vi "Set ATP ComboBox - Single Project Open.vi"(8 "Error In":errorcluster, 10 "Project Name":string, 11 "Project Name ComboBox Ref":refnum<vi>) -> (0 "Error Out":errorcluster)   [LabVIEW 2022 SP3]
doc: "ATP = \"Add to Project?\" drop-down menu"
uses:
  <vilib>/Utility/miscctls.llb/LVFontTypeDef.ctl
panel:
  # "Development\nControls or indicators that are useful for development or testing, but which are not outputs of the VI."
  # "Input\nInputs to the VI"
  # "Output\nOutputs of the VI"
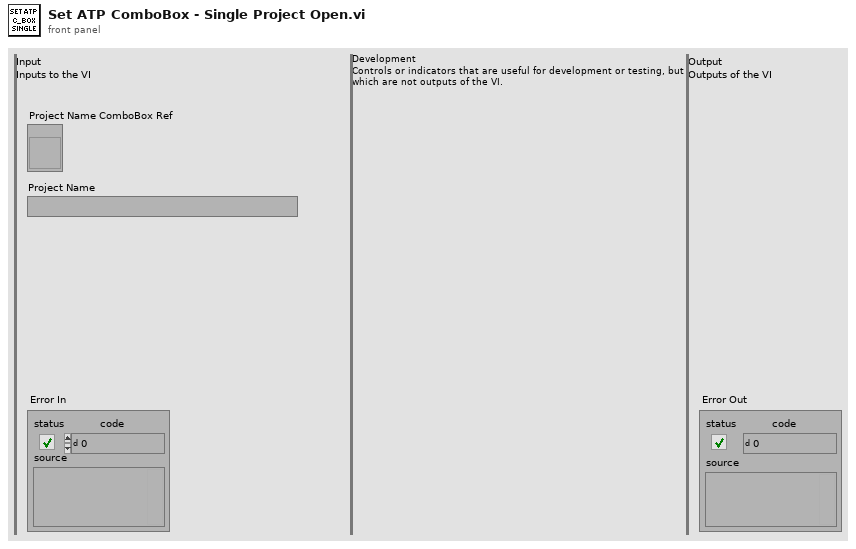
[diagram p1: front panel]
types:
  T1 = typedef "LVFontTypeDef.ctl" = cluster{"Font Name":string, "Size":u16, "Bold":bool, "Italic":bool, "Underline":bool, "Strikeout":bool, "Color":u32}
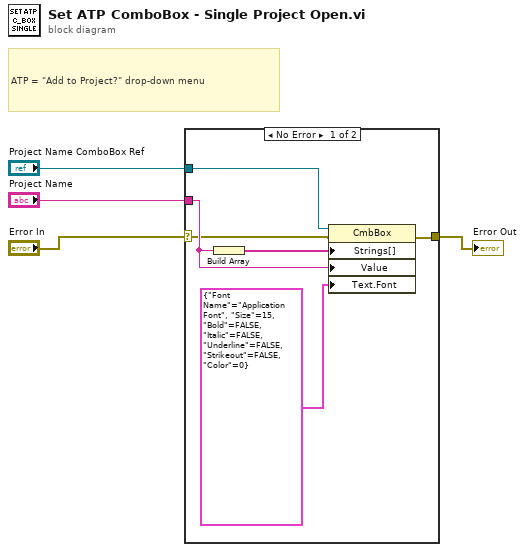
[diagram p0: block diagram]
diagram:
  # "ATP = \"Add to Project?\" drop-down menu"
  n1 = case shown="No Error" "Error In" {
    selector: "Error In" -> [w7 w11]
    tunnel: [w6 w11] -> w3
    tunnel: "Project Name ComboBox Ref" -> [w9 _]
    tunnel: "Project Name" -> [w8 _]
    frame No Error {
      n2 = Build Array(w8) -> (w5:string[])
      n3 = property class="CmbBox"(reference=w9, error in=w7, "Strings[]"=w5, "Value"=w8, "Text.Font"=T1 {"Font Name"="Application Font", "Size"=15, "Bold"=FALSE, "Italic"=FALSE, "Underline"=FALSE, "Strikeout"=FALSE, "Color"=0}) -> (error out=w6:errorcluster)  [unwired: 1 out]
    }
    frame Error {
    }
  }
  "Error Out" <- w3
